vi "Set Parameters GUI.vi"(8 "error in (no error)":errorcluster, 11 "Temp Control in":refnum<class "Temp Control.lvclass">) -> (0 "error out":errorcluster, 3 "Temp Control out":refnum<class "Temp Control.lvclass">)   [LabVIEW 2022 SP3, in "Temp Control.lvclass"]
uses:
  Temp Control.lvclass
  Temp Control.lvclass/Temp Control.ctl
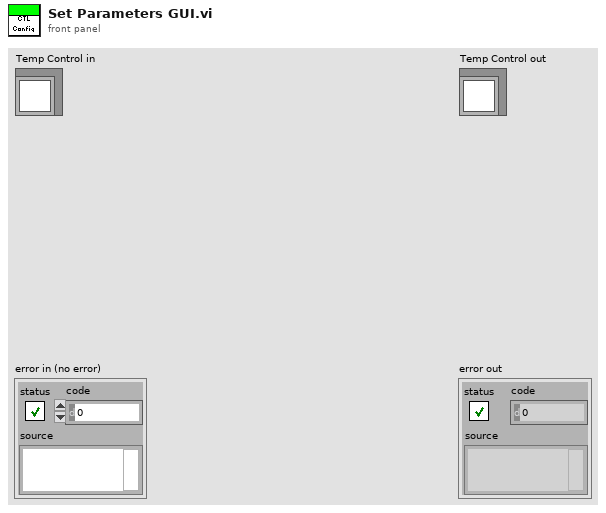
[diagram p1: front panel]
types:
  T1 = typedef "Temp Control.lvclass/Temp Control Sim Settings.ctl" = cluster{"Offsets out":dbl[], "Scaling out":dbl[]}
  T2 = cluster{"Offsets out":dbl[], "Scaling out":dbl[]}
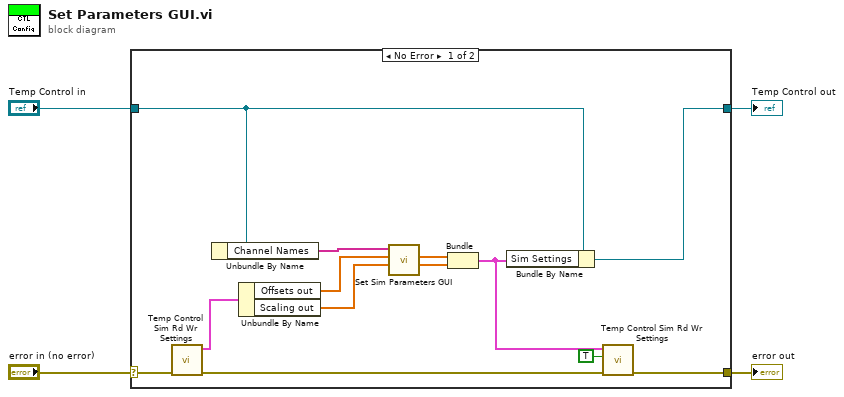
[diagram p0: block diagram]
diagram:
  n1 = case shown="No Error" "error in (no error)" {
    selector: "error in (no error)" -> [w9 w19]
    tunnel: [w11 w19] -> w3
    tunnel: [w14 w18] -> w1
    tunnel: "Temp Control in" -> [w13 w18]
    frame No Error {
      n2 = call "Temp Control Sim Rd Wr Settings.vi"("error in (no error)"=w9) -> ("error out"=w8:errorcluster, "Sim Settings"=w7:T1)  [unwired: 9 in]
      n3 = Unbundle By Name(w13) -> ("Channel Names"=w15:string[])
      n4 = Unbundle By Name(w7) -> ("Offsets out"=w6:dbl[], "Scaling out"=w5:dbl[])
      n5 = call "Set Sim Parameters GUI.vi"("Scaling"=w5, "Offsets"=w6, "Channel"=w15) -> ("Scaling out"=w16:dbl[], "Offsets out"=w17:dbl[])  [unwired: 7 in]
      n6 = Bundle("Offsets out"=w17, "Scaling out"=w16) -> (w12:T2)  [unwired: 1 in]
      n7 = Bundle By Name(cluster=w13, "Sim Settings"=w12) -> (w14:refnum<class "Temp Control.lvclass">)
      n8 = call "Temp Control Sim Rd Wr Settings.vi"("error in (no error)"=w8, "Write? (F:Read)"=TRUE, "Sim Settings"=w12) -> ("error out"=w11:errorcluster)  [unwired: 7 in, 1 out]
    }
    frame Error {
    }
  }
  "error out" <- w3
  "Temp Control out" <- w1
